vi "SetControlValues.vi"(8 "error in (no error)":errorcluster, 11 "Theory in":refnum<class "Theory.lvclass">) -> (0 "error out":errorcluster, 3 "Theory out":refnum<class "Theory.lvclass">)   [LabVIEW 2017, in "Theory.lvclass"]
uses:
  Theory.lvclass
  Theory.lvclass/Theory.ctl
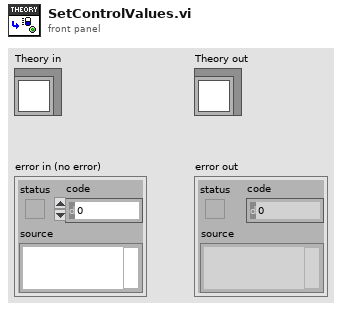
[diagram p1: front panel]
types:
  T1 = typedef "ControlData.ctl" = cluster{"Name":string, "Data":variant}
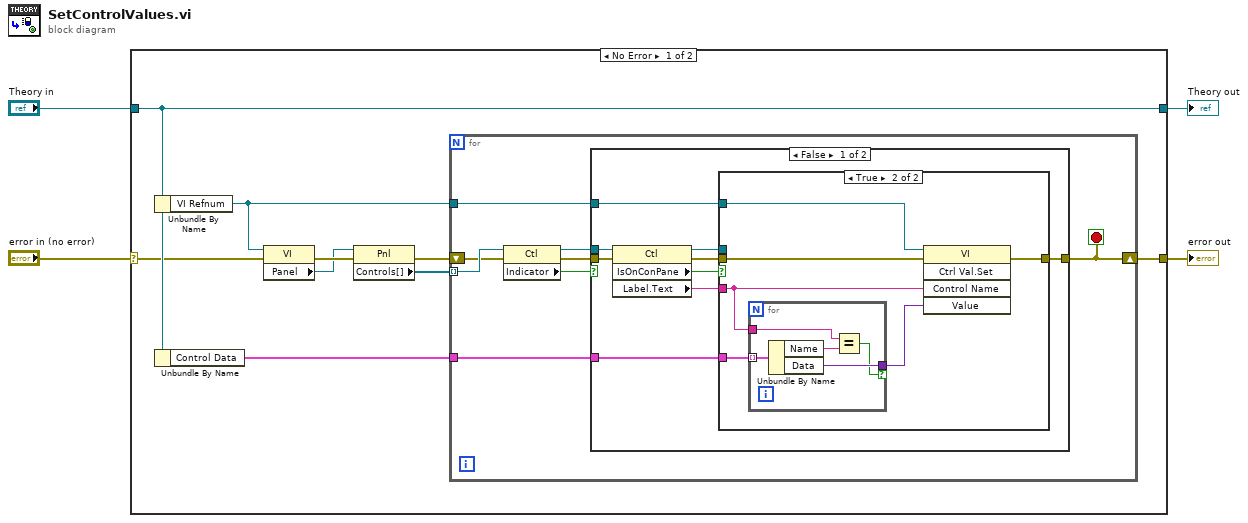
[diagram p0: block diagram]
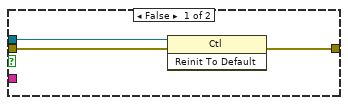
[diagram p2: hidden frame]
diagram:
  n1 = case shown="No Error" "error in (no error)" {
    selector: "error in (no error)" -> [w6 w47]
    tunnel: [w5 w47] -> w3
    tunnel: [w7 w46] -> w1
    tunnel: "Theory in" -> [w7 w46]
    frame No Error {
      n2 = Unbundle By Name(w7) -> ("VI Refnum"=w8:refnum<vi>)
      n3 = Unbundle By Name(w7) -> ("Control Data"=w13:T1[])
      n4 = property class="VI"(reference=w8, error in=w6) -> (error out=w12:errorcluster, "Panel"=w10:refnum<vi>)  [unwired: 1 out]
      n5 = property class="Pnl"(reference=w10, error in=w12) -> (error out=w11:errorcluster, "Controls[]"=w9:refnum<vi>[])  [unwired: 1 out]
      n6 = for {
        tunnel: w8 -> [w20]
        shift-right: [w19] -> w5
        shift-left: w11 -> [w17]
        tunnel: w13 -> [w21]
        tunnel: w9 -> [w18] mode=indexing
        stop <- w19 stop-if-true
        n7 = property class="Ctl"(reference=w18, error in=w17) -> (reference out=w16:refnum<vi>, error out=w15:errorcluster, "Indicator"=w14:bool)
        n8 = case shown="False" w14 {
          tunnel: w21 -> [w28 _]
          tunnel: w20 -> [w25 _]
          tunnel: [w24 w45] -> w19
          tunnel: w16 -> [w23 _]
          tunnel: w15 -> [w22 w45]
          frame False {
            n9 = property class="Ctl"(reference=w23, error in=w22) -> (reference out=w26:refnum<vi>, error out=w29:errorcluster, "IsOnConPane"=w30:bool, "Label.Text"=w27:string)
            n10 = case shown="True" w30 {
              tunnel: [w32 w37] -> w24
              tunnel: w29 -> [w33 w39]
              tunnel: w28 -> [_ w36]
              tunnel: w27 -> [_ w35]
              tunnel: w26 -> [w31 _]
              tunnel: w25 -> [_ w38]
              frame False {
                n11 = invoke class="Ctl" method="Reinit To Default"(reference=w31, error in=w33) -> (error out=w32:errorcluster)  [unwired: 1 in, 2 out]
              }
              frame True {
                n12 = for {
                  tunnel: w36 -> [w44] mode=indexing
                  tunnel: w35 -> [w42]
                  tunnel: [w41] -> w34 if=w40
                  n13 = Unbundle By Name(w44) -> ("Name"=w43:string, "Data"=w41:variant)
                  n14 = Equal?(x=w42, y=w43) -> (x = y?=w40:bool)
                }
                n15 = invoke class="VI" method="Ctrl Val.Set"(reference=w38, error in=w39, "Control Name"=w35, "Value"=w34) -> (error out=w37:errorcluster)  [unwired: 1 in, 4 out]
              }
            }
          }
          frame True {
          }
        }
      }
    }
    frame Error {
    }
  }
  "error out" <- w3
  "Theory out" <- w1
